vi "Stop Core.vi"(10 "final error code":i32, 11 "Main_UI in":refnum<class "Main_UI.lvclass">) -> (3 "Main_UI out":refnum<class "Main_UI.lvclass">)   [LabVIEW 2020, in "Main_UI.lvlib" / "Main_UI.lvclass"]
doc: "(<B>Filename</B>: Actor Framework.lvlib:Actor.lvclass:Stop Core.vi)\n\nDefines what the actor does before it stops. Use the <B>final error code</B> input to determine whether the actor shut down in response to an error.\n\nBy default, this method passes the Stop message along to all auto-stop nested actors. A descendant class may override this method to define additional behavior, such as shutting down any processes the actor initiated in its override of the Actor Core method."
uses:
  Main_UI.lvclass
  Main_UI.lvclass/Main_UI.ctl
  <vilib>/ActorFramework/Actor/Actor.lvclass
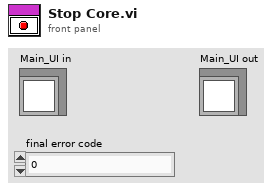
[diagram p1: front panel]
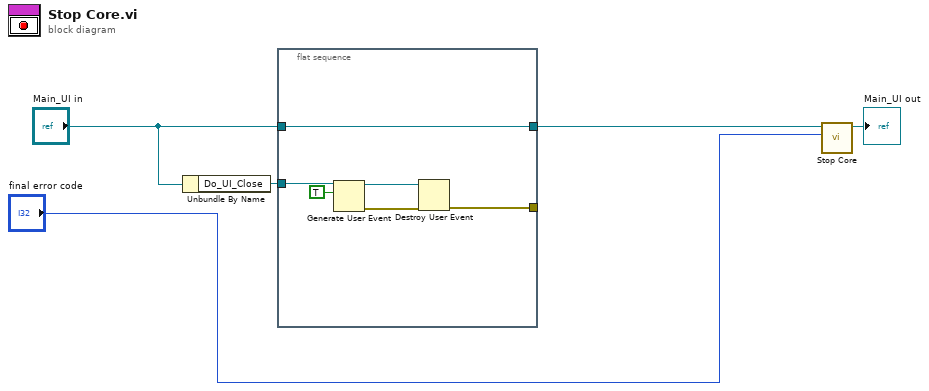
[diagram p0: block diagram]
diagram:
  n1 = Unbundle By Name("Main_UI in") -> ("Do_UI_Close"=w4:refnum<user-event>)
  n2 = flat-sequence {
    tunnel: w4 -> [w11]
    tunnel: "Main_UI in" -> [w7]
    tunnel: [w7] -> w1
    tunnel: [w6] -> _
    frame #0 {
      n3 = Generate User Event(user event=w11, event data cluster=TRUE ("event data")) -> (user event out=w9:refnum<user-event>, error out=w8:errorcluster)  [unwired: 2 in]
      n4 = Destroy User Event(user event=w9, error in=w8) -> (error out=w6:errorcluster)
    }
  }
  n5 = call-parent "Stop Core.vi"("final error code"="final error code", "Actor in"=w1) -> ("Actor out"=→"Main_UI out":refnum<class "Main_UI.lvclass">)  [unwired: 9 in]
